vi "Main.vi"(11 "Module Admin":refnum<class "Delacor_lib_QMH_Module Admin.lvclass">) -> ()   [LabVIEW 2020, in "Configuration.lvlib"]
doc: "This template is based off of the Queued Message Handler design pattern and the Queued Message Handler project template that ships with LabVIEW.\n\nThe main difference is that the queue is private to this module and communication between modules is performed via Broadcast and Request events.\n\nRequest events are wrapped in public API methods and are handled in the Event Handling Loop (EHL) of this VI. Any module can register for Broadcast events sent by this module. The EHL generates messages based on user interface actions.\n\nThe Message Handling Loop (MHL) processes messages generated by the EHL, or by other messages. The messages are string values, so new messages can be added easily to the Message Cases case structure in the MHL. Each message cluster can also provide an optional value for Message Data, which is a variant that can be converted to whatever message-specific data is required.\n_____\nBased on Delacor QMH Project Template 5.0.0.82."
uses:
  Configuration.lvlib
  <vilib>/Delacor/Delacor QMH/Libraries/Module Admin_class/Delacor_lib_QMH_Module Admin.lvclass
  Module Data--cluster.ctl
  Stop Argument--cluster.ctl
  <vilib>/Delacor/Delacor QMH/Libraries/Message Queue_class/Delacor_lib_QMH_Message Queue.lvclass/Delacor_lib_QMH_Message Queue.ctl
  SQLITE Inventory/Invetory Data Type.ctl
  <vilib>/Utility/miscctls.llb/LVPointTypeDef.ctl
  <vilib>/Delacor/Delacor QMH/Libraries/Module Admin_class/Delacor_lib_QMH_Module Admin.lvclass/Delacor_lib_QMH_Module Admin.ctl
  TypeDefinitions/CurrencyEnum.ctl
  <vilib>/Delacor/Delacor QMH/Libraries/Message Queue_class/Delacor_lib_QMH_Enqueue Message (Single).vi
  <vilib>/Delacor/Delacor QMH/Libraries/Module Admin_class/Delacor_lib_QMH_Get External Launch.vi
  <vilib>/Utility/error.llb/Error Cluster From Error Code.vi
  <vilib>/ErrorRing/Error Ring.xnode
  <vilib>/Delacor/Delacor QMH/Libraries/Message Queue_class/Delacor_lib_QMH_Message Queue.lvclass
  SQLITE Inventory/SQLITE Inventory.lvlib
  Product Selecting Pane/Product Selecting Pane.lvlib
  Money Control Pane/Money Control Pane.lvlib
  Config Files Management/Config File Management.lvlib
panel:
  in  "Change Currency":bool
  in  "Coin Management":T1
  in  "Inventory Management":T2(tab)
  in  "Add Product":bool
  in  "Quantity":dbl
  in  "Price":dbl
  in  "Product Name":string
  in  "Change Stock":bool
  in  "Add to stock":bool
  in  "Stock":u32
  in  "Product UI":u16(ring) items=["Cheetos", "Cheetos Puff", "Doritos 3D", "Doritos Incognita", "Doritos Nacho", "Gomilokas", "Takis Verde"]
  in  "Update all price":bool
  in  "Convertion Ratio":dbl
  in  "Update single price":bool
  in  "New Price":dbl
  in  "Product UP":u16(ring) items=["Cheetos", "Cheetos Puff", "Doritos 3D", "Doritos Incognita", "Doritos Nacho", "Gomilokas", "Takis Verde"]
  in  "Product D":u16(ring) items=["Cheetos", "Cheetos Puff", "Doritos 3D", "Doritos Incognita", "Doritos Nacho", "Gomilokas", "Takis Verde"]
  in  "Delete":bool
  out "error out":errorcluster
  # "General Settings"
  # "1 of old currency is equal to"
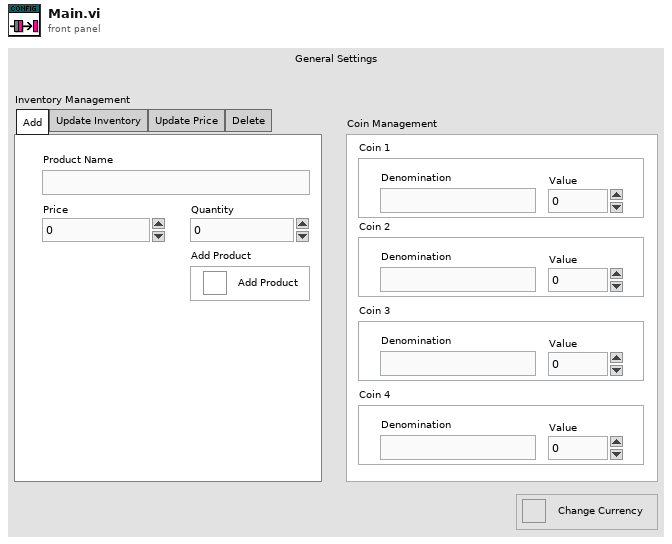
[diagram p1: front panel]
types:
  T1 = cluster{"Coin 1":cluster{"Denomination":string, "Value":dbl}, "Coin 2":cluster{"Denomination":string, "Value":dbl}, "Coin 3":cluster{"Denomination":string, "Value":dbl}, "Coin 4":cluster{"Denomination":string, "Value":dbl}}
  T2 = enum32{"Add", "Update Inventory", "Update Price", "Delete"}
  T3 = typedef "Configuration.lvlib/Request Events--cluster.ctl" = cluster{"Stop Module":refnum<user-event>, "Show Panel":refnum<user-event>, "Hide Panel":refnum<user-event>, "Get Module Execution Status":refnum<user-event>, "Show Diagram":refnum<user-event>}
  T4 = typedef "Configuration.lvlib/Module Data--cluster.ctl" = cluster{"Status":string, "Products":string[], "Ref Array":refnum<vi>[], "Product UI":string, "Product UP":string, "Product D":string, "Stock":u32}
  T5 = enum32{"invalid lock state", "Not Locked", "Locked (No Password)", "Password-protected"}
  T6 = typedef "Configuration.lvlib/Stop Argument--cluster.ctl" = cluster{"Origin":string, "Exit via Stop Module Req?":bool, "Wait for Module to stop?":bool}
  T7 = typedef "Invetory Data Type.ctl" = cluster{"Name":string, "Price":dbl, "Stock":dbl}
  T8 = typedef "LVPointTypeDef.ctl" = cluster{"Horizontal":i16, "Vertical":i16}
  T9 = enum32{"Invalid", "Standard", "Closed", "Hidden", "Minimized", "Maximized"}
  T10 = typedef "CurrencyEnum.ctl" = enum16{"USD", "MXN", "EUR", "GBP"}
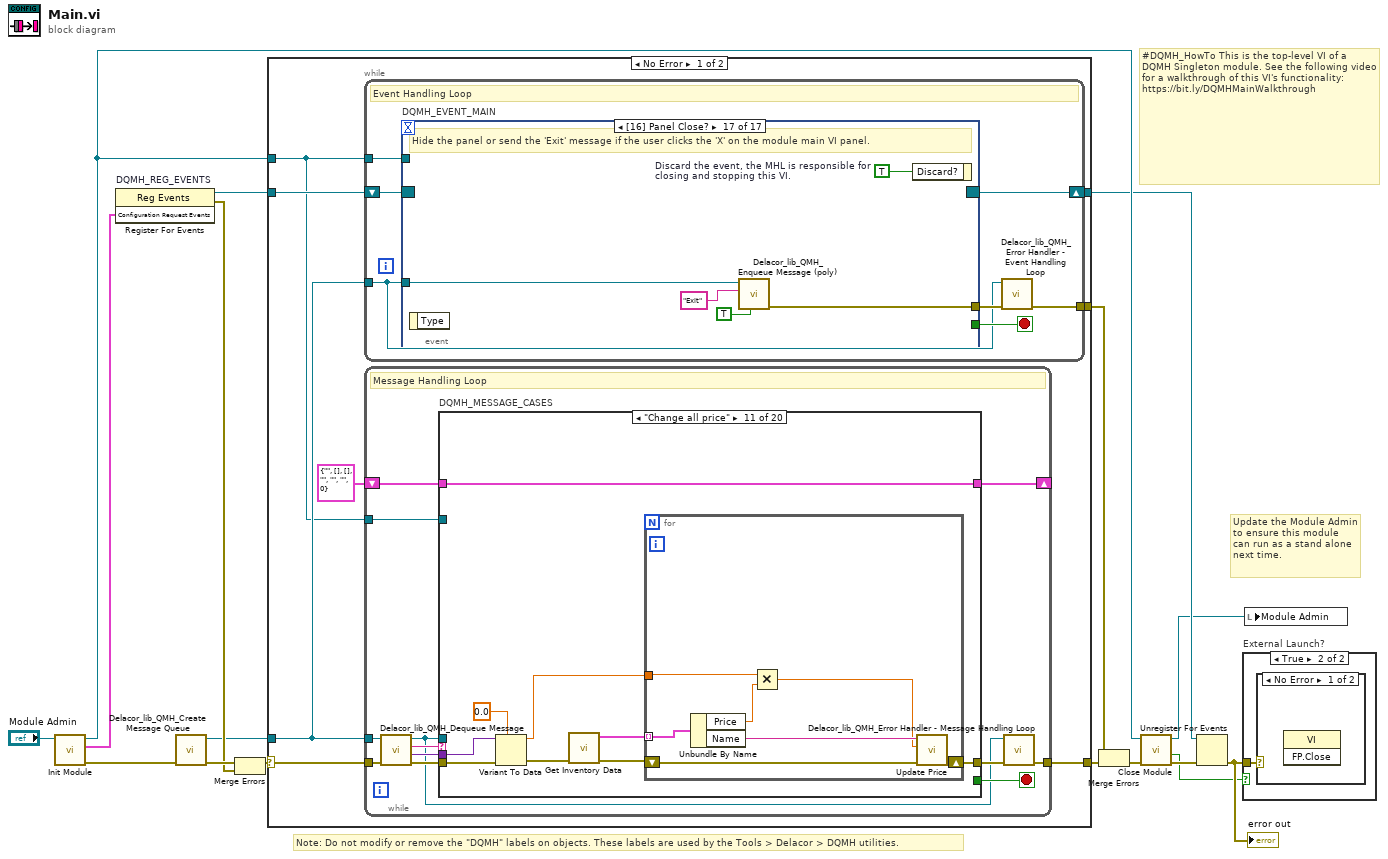
[diagram p0: block diagram]
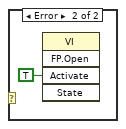
[diagram p3: hidden frame]
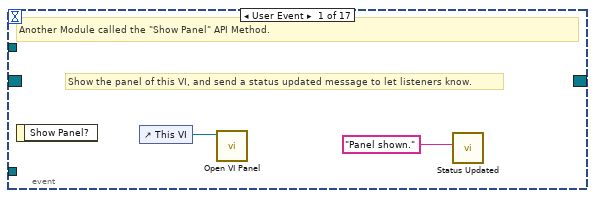
[diagram p4: hidden frame]
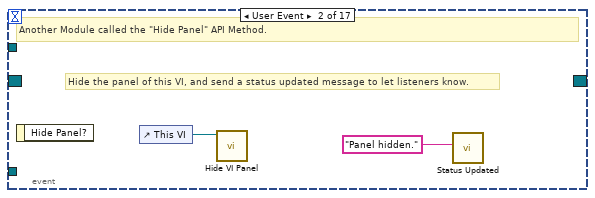
[diagram p5: hidden frame]
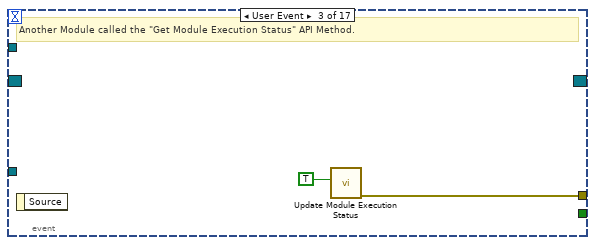
[diagram p6: hidden frame]
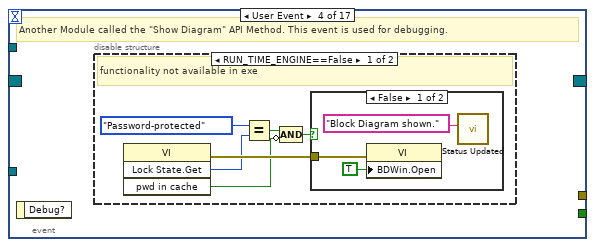
[diagram p7: hidden frame]
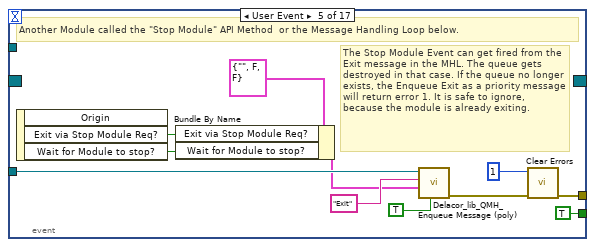
[diagram p10: hidden frame]
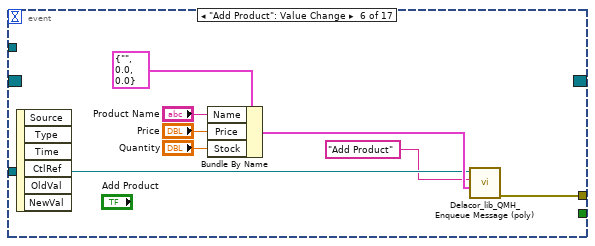
[diagram p11: hidden frame]
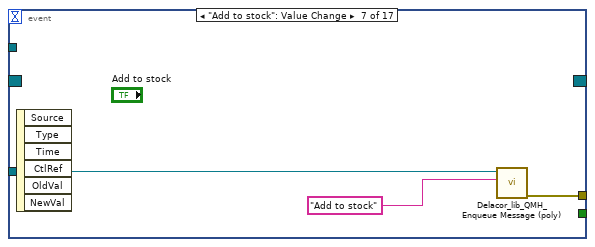
[diagram p12: hidden frame]
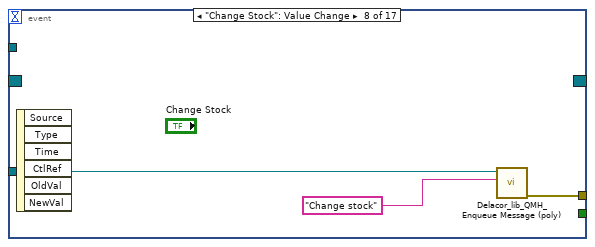
[diagram p13: hidden frame]
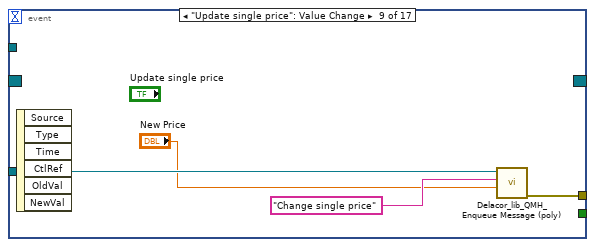
[diagram p14: hidden frame]
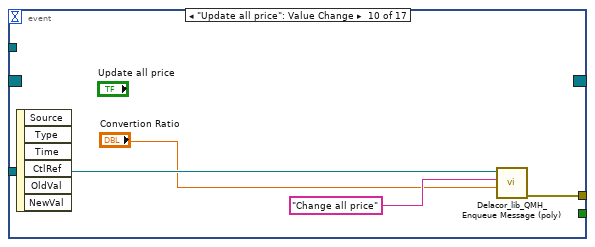
[diagram p15: hidden frame]
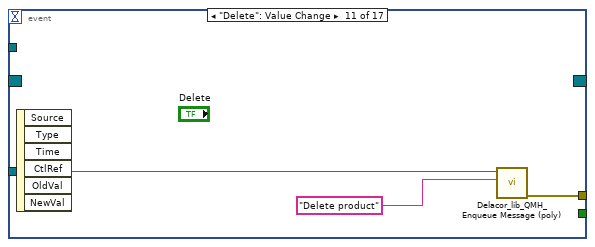
[diagram p16: hidden frame]
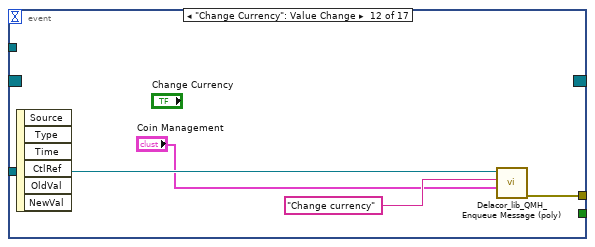
[diagram p17: hidden frame]
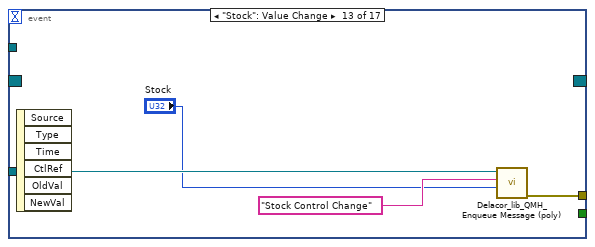
[diagram p18: hidden frame]
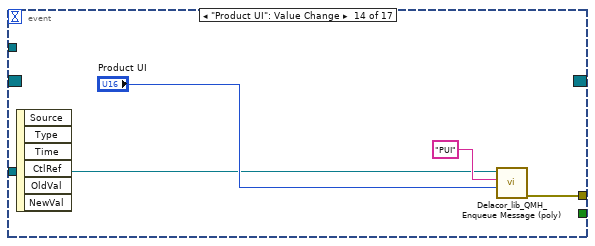
[diagram p19: hidden frame]
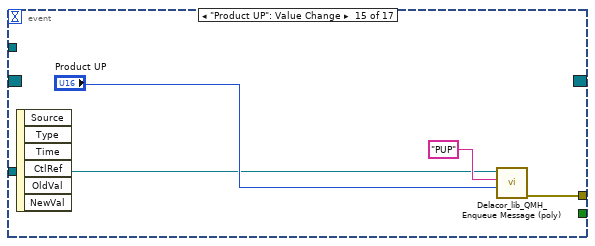
[diagram p20: hidden frame]
diagram:
  # "#DQMH_HowTo This is the top-level VI of a DQMH Singleton module. See the following video for a walkthrough of this VI's functionality: https://bit.ly/DQMHMainWalkthrough"
  # "Note: Do not modify or remove the \"DQMH\" labels on objects. These labels are used by the Tools > Delacor > DQMH utilities."
  # "Update the Module Admin to ensure this module can run as a stand alone next time."
  n1 = call "Init Module.vi"("Singleton Module Admin in"="Module Admin") -> ("error out"=w16:errorcluster, "Configuration Request Events"=w5:T3, "Singleton Module Admin out"=w8:refnum<class "Delacor_lib_QMH_Module Admin.lvclass">)  [unwired: 8 in]
  n2 = register-events "DQMH_REG_EVENTS"(w5) -> (reference out=w6:refnum<event-registration>, error out=w9:errorcluster)  [unwired: 2 in]
  n3 = call <vilib>:"Delacor_lib_QMH_Create Message Queue.vi"("error in (no error)"=w16) -> ("error out"=w11:errorcluster, "Message Queue"=w4:refnum<class "Delacor_lib_QMH_Message Queue.lvclass">)  [unwired: 9 in]
  n4 = Merge Errors(w11, w9) -> (w10:errorcluster)
  n5 = case shown="No Error" w10 {
    selector: w10 -> [w23 w329]
    tunnel: [w25 w328] -> w17
    tunnel: [w22 w334] -> w7
    tunnel: w6 -> [w20 w334]
    tunnel: w4 -> [w19 w327]
    tunnel: [w24 _] -> w14
    tunnel: w8 -> [w18 w330]
    frame No Error {
      n6 = while {
        tunnel: w19 -> [w26]
        shift-right: [w29] -> w22
        shift-left: w20 -> [w30]
        tunnel: [w31] -> w24
        tunnel: w18 -> [w27]
        stop <- w28 stop-if-true
        # "Event Handling Loop"
        n7 = event "DQMH_EVENT_MAIN" shown="[16] Panel Close?" {
          selector: w30 -> [_ _ _ _ _ _ _ _ _ _ _ _ _ _ _ _ _]
          dyn-events: [_ _ _ _ _ _ _ _ _ _ _ _ _ _ _ _ _] -> w29
          timeout: _ -> [_ _ _ _ _ _ _ _ _ _ _ _ _ _ _ _ _]
          tunnel: [_ _ _ _ TRUE ("Discard?") _ _ _ _ _ _ _ _ _ _ _ _] -> w28
          tunnel: w26 -> [_ _ _ _ w54 w60 w67 w70 w74 w78 w81 w85 w89 w92 w96 w100 w106]
          tunnel: [_ _ w38 _ w57 w66 w69 w72 w76 w80 w83 w87 w91 w95 w99 w103 w108] -> w32
          tunnel: w27 -> [_ _ _ _ _ _ _ _ _ _ _ _ _ _ _ _ _]
          event User Event {
            # "Show the panel of this VI, and send a status updated message to let listeners know."
            # "Another Module called the \"Show Panel\" API Method."
            n8 = event-data() -> ()  [unwired: 1 in, 1 out]
            n9 = control-ref of="This VI"() -> (w34:refnum<vi>)
            n10 = call "Open VI Panel.vi"("VI"=w34) -> ()  [unwired: 10 in, 1 out]
            n11 = call "Status Updated.vi"("Status"="Panel shown." ("format string")) -> ()  [unwired: 10 in, 1 out]
          }
          event User Event {
            # "Hide the panel of this VI, and send a status updated message to let listeners know."
            # "Another Module called the \"Hide Panel\" API Method."
            n12 = event-data() -> ()  [unwired: 1 in, 1 out]
            n13 = control-ref of="This VI"() -> (w36:refnum<vi>)
            n14 = call "Hide VI Panel.vi"("VI"=w36) -> ()  [unwired: 10 in, 1 out]
            n15 = call "Status Updated.vi"("Status"="Panel hidden." ("format string")) -> ()  [unwired: 10 in, 1 out]
          }
          event User Event {
            # "Another Module called the \"Get Module Execution Status\" API Method."
            n16 = event-data() -> ()  [unwired: 1 in, 1 out]
            n17 = call "Update Module Execution Status.vi"("Running?"=TRUE) -> ("error out"=w38:errorcluster)  [unwired: 10 in]
          }
          event User Event {
            # "Another Module called the \"Show Diagram\" API Method. This event is used for debugging."
            n18 = event-data() -> ()  [unwired: 1 in, 1 out]
            n19 = disable-structure shown="RUN_TIME_ENGINE==False" {
              frame condition #0 (active) {
                # "functionality not available in exe"
                n20 = invoke class="VI" method="Lock State.Get"() -> (error out=w44:errorcluster, "Get Lock State"=w43:T5, "pwd in cache"=w40:bool)  [unwired: 4 in, 1 out]
                n21 = Equal?(x=T5."Password-protected", y=w43) -> (x = y?=w41:bool)
                n22 = Compound Arithmetic op=AND(w41, invert w40) -> (w39:bool)
                n23 = case shown="False" w39 {
                  tunnel: w44 -> [w47 _]
                  frame False {
                    n24 = property class="VI"(error in=w47, "BDWin.Open"=TRUE ("Block Diagram Window:Open")) -> ()  [unwired: 1 in, 2 out]
                    n25 = call "Status Updated.vi"("Status"="Block Diagram shown." ("format string")) -> ()  [unwired: 10 in, 1 out]
                  }
                  frame True {
                    # "Password-protected VI, and the password is not in the cache. Do not show the diagram."
                  }
                }
              }
              frame condition #1 {
              }
            }
          }
          event User Event {
            # "The Stop Module Event can get fired from the Exit message in the MHL. The queue gets destroyed in that case. If the queue no longer exists, the Enqueue Exit as a priority message will return error 1. It is safe to ignore, because the module is already exiting."
            # "Another Module called the \"Stop Module\" API Method  or the Message Handling Loop below."
            n26 = event-data() -> ("Exit via Stop Module Req?"=w50:bool, "Wait for Module to stop?"=w49:bool)  [unwired: 1 in, 1 out]
            n27 = Bundle By Name(cluster=T6 {"Origin"="", "Exit via Stop Module Req?"=FALSE, "Wait for Module to stop?"=FALSE} ("Stop Argument"), "Exit via Stop Module Req?"=w50, "Wait for Module to stop?"=w49) -> (w48:T6)
            n28 = call-poly <vilib>:"Delacor_lib_QMH_Enqueue Message (poly).vi"("Priority Message? (F)"=TRUE, "Message Data"=w48, "Message"="Exit", "Message Queue in"=w54) -> ("error out"=w58:errorcluster)  [unwired: 6 in, 1 out]
            n29 = call <vilib>:"Clear Errors.vi"("error in (no error)"=w58, "specific error code to clear (0: all)"=1) -> ("error out"=w57:errorcluster)  [unwired: 4 in, 1 out]
          }
          event "Add Product": Value Change {
            n30 = event-data() -> ()  [unwired: 1 in, 6 out]
            n31 = Bundle By Name(cluster=T7 {"Name"="", "Price"=0.0, "Stock"=0.0} ("Cluster"), "Name"="Product Name", "Price"="Price", "Stock"="Quantity") -> (w61:T7)
            n32 = call-poly <vilib>:"Delacor_lib_QMH_Enqueue Message (poly).vi"("Message Data"=w61, "Message"="Add Product", "Message Queue in"=w60) -> ("error out"=w66:errorcluster)  [unwired: 7 in, 1 out]
          }
          event "Add to stock": Value Change {
            n33 = event-data() -> ()  [unwired: 1 in, 6 out]
            n34 = call-poly <vilib>:"Delacor_lib_QMH_Enqueue Message (poly).vi"("Message"="Add to stock", "Message Queue in"=w67) -> ("error out"=w69:errorcluster)  [unwired: 8 in, 1 out]
          }
          event "Change Stock": Value Change {
            n35 = event-data() -> ()  [unwired: 1 in, 6 out]
            n36 = call-poly <vilib>:"Delacor_lib_QMH_Enqueue Message (poly).vi"("Message"="Change stock", "Message Queue in"=w70) -> ("error out"=w72:errorcluster)  [unwired: 8 in, 1 out]
          }
          event "Update single price": Value Change {
            n37 = event-data() -> ()  [unwired: 1 in, 6 out]
            n38 = call-poly <vilib>:"Delacor_lib_QMH_Enqueue Message (poly).vi"("Message Data"="New Price", "Message"="Change single price", "Message Queue in"=w74) -> ("error out"=w76:errorcluster)  [unwired: 7 in, 1 out]
          }
          event "Update all price": Value Change {
            n39 = event-data() -> ()  [unwired: 1 in, 6 out]
            n40 = call-poly <vilib>:"Delacor_lib_QMH_Enqueue Message (poly).vi"("Message Data"="Convertion Ratio", "Message"="Change all price", "Message Queue in"=w78) -> ("error out"=w80:errorcluster)  [unwired: 7 in, 1 out]
          }
          event "Delete": Value Change {
            n41 = event-data() -> ()  [unwired: 1 in, 6 out]
            n42 = call-poly <vilib>:"Delacor_lib_QMH_Enqueue Message (poly).vi"("Message"="Delete product", "Message Queue in"=w81) -> ("error out"=w83:errorcluster)  [unwired: 8 in, 1 out]
          }
          event "Change Currency": Value Change {
            n43 = event-data() -> ()  [unwired: 1 in, 6 out]
            n44 = call-poly <vilib>:"Delacor_lib_QMH_Enqueue Message (poly).vi"("Message Data"="Coin Management", "Message"="Change currency", "Message Queue in"=w85) -> ("error out"=w87:errorcluster)  [unwired: 7 in, 1 out]
          }
          event "Stock": Value Change {
            n45 = event-data() -> ()  [unwired: 1 in, 6 out]
            n46 = call-poly <vilib>:"Delacor_lib_QMH_Enqueue Message (poly).vi"("Message Data"="Stock", "Message"="Stock Control Change", "Message Queue in"=w89) -> ("error out"=w91:errorcluster)  [unwired: 7 in, 1 out]
          }
          event "Product UI": Value Change {
            n47 = event-data() -> ()  [unwired: 1 in, 6 out]
            n48 = call-poly <vilib>:"Delacor_lib_QMH_Enqueue Message (poly).vi"("Message Data"="Product UI", "Message"="PUI", "Message Queue in"=w92) -> ("error out"=w95:errorcluster)  [unwired: 7 in, 1 out]
          }
          event "Product UP": Value Change {
            n49 = event-data() -> ()  [unwired: 1 in, 6 out]
            n50 = call-poly <vilib>:"Delacor_lib_QMH_Enqueue Message (poly).vi"("Message Data"="Product UP", "Message"="PUP", "Message Queue in"=w96) -> ("error out"=w99:errorcluster)  [unwired: 7 in, 1 out]
          }
          event "Product D": Value Change {
            n51 = event-data() -> ()  [unwired: 1 in, 6 out]
            n52 = call-poly <vilib>:"Delacor_lib_QMH_Enqueue Message (poly).vi"("Message Data"="Product D", "Message"="PD", "Message Queue in"=w100) -> ("error out"=w103:errorcluster)  [unwired: 7 in, 1 out]
          }
          event Panel Close? {
            w107 = TRUE  # Discard the event, the MHL is responsible for closing and stopping this VI.
            # "Hide the panel or send the 'Exit' message if the user clicks the 'X' on the module main VI panel."
            n53 = event-data() -> ()  [unwired: 1 in, 1 out]
            n54 = call-poly <vilib>:"Delacor_lib_QMH_Enqueue Message (poly).vi"("Priority Message? (F)"=TRUE, "Message"="Exit", "Message Queue in"=w106) -> ("error out"=w108:errorcluster)  [unwired: 7 in, 1 out]
            n55 = event-data("Discard?"=w107) -> ()  [unwired: 1 in, 1 out]
          }
        }
        n56 = call-dynamic "Delacor_lib_QMH_Error Handler - Event Handling Loop.vi"("error in (no error)"=w32, "Message Queue in"=w26) -> ("dup error in"=w31:errorcluster)  [unwired: 8 in, 1 out]
      }
      n57 = while {
        tunnel: w19 -> [w111]
        shift-right: [w115] -> _
        shift-left: T4 {"Status"="", "Products"=[], "Ref Array"=[], "Product UI"="", "Product UP"="", "Product D"="", "Stock"=0} ("Data Cluster") -> [w116]
        tunnel: w23 -> [w119]
        tunnel: [w117] -> w25
        tunnel: w18 -> [w109]
        stop <- w114 stop-if-true
        # "Message Handling Loop"
        n58 = call-dynamic "Delacor_lib_QMH_Dequeue Message.vi"("error in (no error)"=w119, "Message Queue in"=w111) -> ("error out"=w118:errorcluster, "Message Data"=w112:variant, "Message"=w113:string, "Message Queue out"=w110:refnum<class "Delacor_lib_QMH_Message Queue.lvclass">)  [unwired: 6 in]
        n59 = case "DQMH_MESSAGE_CASES" shown="\"Change all price\"" w113 {
          selector: w113 -> [_ _ _ _ _ _ _ _ _ _ _ _ _ _ _ _ _ _ _ w314]
          tunnel: w110 -> [w125 _ _ _ _ _ _ _ _ _ _ _ w245 _ _ _ _ w283 w306 _]
          tunnel: w118 -> [w145 w153 w167 w176 w185 w187 w199 w207 w210 w221 w229 w244 w254 w262 w265 w267 w272 w290 w312 w316]
          tunnel: [w127 w152 w166 w175 w184 w186 w198 w206 w211 w214 w223 w242 w247 w262 w264 w267 w271 w286 w309 w317] -> w120
          tunnel: w116 -> [w135 w151 w161 w170 w179 w195 w200 w208 w212 w220 w230 w243 w253 w261 w263 w266 w269 w285 w305 w315]
          tunnel: [w134 w149 w164 w173 w182 w195 w200 w208 w212 w220 w230 w239 w253 w261 w263 w266 w269 w285 w305 w315] -> w115
          tunnel: [_ _ _ _ _ _ _ _ _ _ _ _ _ _ _ _ _ _ w304 _] -> w114
          tunnel: w112 -> [_ _ w165 w174 w183 _ _ w203 _ w218 w228 w241 w252 _ _ _ _ w284 w303 _]
          tunnel: w109 -> [w136 _ _ _ _ _ _ _ _ _ _ _ _ _ _ _ _ w282 w298 _]
          frame "Initialize" {
            # "Initialize - Any operation that needs to be done before the module can receive messages. Synchronize Caller Events.vi will inform Start Module.vi that the module has launched and is ready to receive messages. Module Did Init.vi will broadcast that the module initialized."
            n60 = call "Synchronize Caller Events.vi"("error in (no error)"=w145, "Singleton Module Admin in"=w136) -> ("error out"=w144:errorcluster, "Singleton Module Admin out"=w131:refnum<class "Delacor_lib_QMH_Module Admin.lvclass">)  [unwired: 8 in]
            n61 = property class="Module Admin"(reference=w131) -> ("Accessors:External Launch"=w140:bool)  [unwired: 1 in, 2 out]
            n62 = control-ref of="Product D"() -> (w124:refnum<vi>)
            n63 = control-ref of="Product UP"() -> (w123:refnum<vi>)
            n64 = control-ref of="Product UI"() -> (w122:refnum<vi>)
            n65 = Build Array(w124, w123, w122) -> (w121:refnum<vi>[])
            n66 = Select(t=T9."Hidden" ("State"), s=w140, f=T9."Standard" ("State")) -> (s? t:f=w137:T9)
            n67 = call "Module Name--constant.vi"() -> ("Module Name"=w132:string)  [unwired: 11 in]
            n68 = call "Module Name--constant.vi"() -> ("Module Name"=w143:string)  [unwired: 11 in]
            n69 = call "Module Did Init.vi"("error in (no error)"=w144, "Initialized?"=TRUE, "Origin"=w132) -> ("error out"=w128:errorcluster)  [unwired: 8 in]
            n70 = property class="VI"("Front Panel.Title"=w143) -> (reference out=w142:refnum<vi>, error out=w147:errorcluster)  [unwired: 2 in]
            n71 = invoke class="VI" method="FP.Open"(reference=w142, error in=w147, "State"=w137) -> (reference out=w141:refnum<vi>, error out=w146:errorcluster)  [unwired: 2 in, 3 out]
            n72 = Bundle By Name(cluster=w135, "Status"="Initial Message" ("Initial Message"), "Ref Array"=w121) -> (w134:T4)
            n73 = call-poly <vilib>:"Delacor_lib_QMH_Enqueue Message (poly).vi"("error in (no error)"=w128, "Message"="Update DB", "Message Queue in"=w125) -> ("error out"=w127:errorcluster)  [unwired: 7 in, 1 out]
            n74 = invoke class="VI" method="FP.Center"(reference=w141, error in=w146) -> ()  [unwired: 1 in, 3 out]
            n75 = property on="Pane" class="Pane"("Origin"=T8 {"Horizontal"=0, "Vertical"=0}) -> ()  [unwired: 2 in, 2 out]
          }
          frame "Update DB" {
            # "Update product Controls when DB products has been modified"
            n76 = call "Get Inventory Data.vi"("error in (no error)"=w153) -> ("error out"=w152:errorcluster, "Array"=w154:T7[])  [unwired: 9 in]
            n77 = Unbundle By Name(w151) -> ("Ref Array"=w150:refnum<vi>[])
            n78 = for {
              tunnel: w154 -> [w158] mode=indexing
              tunnel: [w157] -> w148 mode=indexing
              n79 = Unbundle By Name(w158) -> ("Name"=w157:string)
            }
            n80 = for {
              tunnel: w148 -> [w156]
              tunnel: w150 -> [w155] mode=indexing
              n81 = property class="Ring (strict)"(reference=w155, "Strings []"=w156) -> ()  [unwired: 1 in, 2 out]
            }
            n82 = Bundle By Name(cluster=w151, "Products"=w148) -> (w149:T4)
          }
          frame "PUI" {
            n83 = Variant To Data(error in=w167, type=u16 0, Variant=w165) -> (data=w162:u16, error out=w166:errorcluster)
            n84 = Unbundle By Name(w161) -> ("Products"=w160:string[])
            n85 = Index Array(array=w160, index=w162) -> (element=w159:string)
            n86 = Bundle By Name(cluster=w161, "Product UI"=w159) -> (w164:T4)
          }
          frame "PUP" {
            n87 = Variant To Data(error in=w176, type=u16 0, Variant=w174) -> (data=w171:u16, error out=w175:errorcluster)
            n88 = Unbundle By Name(w170) -> ("Products"=w169:string[])
            n89 = Index Array(array=w169, index=w171) -> (element=w168:string)
            n90 = Bundle By Name(cluster=w170, "Product UP"=w168) -> (w173:T4)
          }
          frame "PD" {
            n91 = Variant To Data(error in=w185, type=u16 0, Variant=w183) -> (data=w180:u16, error out=w184:errorcluster)
            n92 = Unbundle By Name(w179) -> ("Products"=w178:string[])
            n93 = Index Array(array=w178, index=w180) -> (element=w177:string)
            n94 = Bundle By Name(cluster=w179, "Product D"=w177) -> (w182:T4)
          }
          frame "Add to stock" {
            n95 = Unbundle By Name(w195) -> ("Product UI"=w194:string, "Stock"=w190:u32)
            n96 = call "Get Product Info.vi"("error in (no error)"=w187, "Name"=w194) -> ("error out"=w188:errorcluster, "Product Info"=w193:T7)  [unwired: 7 in, 1 out]
            n97 = Unbundle By Name(w193) -> ("Name"=w192:string, "Stock"=w191:dbl)
            n98 = Add(x=w191, y=w190) -> (x+y=w189:dbl)
            n99 = call "Update Stock.vi"("error in (no error)"=w188, "Stock"=w189, "Name"=w192) -> ("error out"=w186:errorcluster)  [unwired: 8 in]
          }
          frame "Change stock" {
            n100 = Unbundle By Name(w200) -> ("Product UI"=w196:string, "Stock"=w197:u32)
            n101 = call "Update Stock.vi"("error in (no error)"=w199, "Stock"=w197, "Name"=w196) -> ("error out"=w198:errorcluster)  [unwired: 8 in]
          }
          frame "Change single price" {
            n102 = Unbundle By Name(w208) -> ("Product UP"=w205:string)
            n103 = Variant To Data(error in=w207, type=0.0 ("New Price"), Variant=w203) -> (data=w201:dbl, error out=w204:errorcluster)
            n104 = call "Update Price.vi"("error in (no error)"=w204, "Price"=w201, "Name"=w205) -> ("error out"=w206:errorcluster)  [unwired: 8 in]
          }
          frame "Delete product" {
            n105 = Unbundle By Name(w212) -> ("Product D"=w209:string)
            n106 = call "Delete Product.vi"("error in (no error)"=w210, "Name"=w209) -> ("error out"=w211:errorcluster)  [unwired: 9 in]
          }
          frame "Change currency" {
            n107 = Variant To Data(error in=w221, type=T1 {"Coin 1"={"Denomination"="", "Value"=0.0}, "Coin 2"={"Denomination"="", "Value"=0.0}, "Coin 3"={"Denomination"="", "Value"=0.0}, "Coin 4"={"Denomination"="", "Value"=0.0}} ("Coin Management"), Variant=w218) -> (data=w216:T1, error out=w219:errorcluster)
            n108 = Cluster To Array(cluster=w216) -> (array=w215:cluster{"Denomination":string, "Value":dbl}[])
            n109 = call "Change Currency.vi"("Coin"=w215) -> ("error out"=w213:errorcluster)  [unwired: 10 in]
            n110 = Merge Errors(w213, w219) -> (w214:errorcluster)
          }
          frame "Change all price" {
            n111 = Variant To Data(error in=w229, type=0.0 ("New Price"), Variant=w228) -> (data=w222:dbl, error out=w225:errorcluster)
            n112 = call "Get Inventory Data.vi"("error in (no error)"=w225) -> ("error out"=w224:errorcluster, "Array"=w226:T7[])  [unwired: 9 in]
            n113 = for {
              tunnel: w226 -> [w235] mode=indexing
              shift-right: [w236] -> w223
              shift-left: w224 -> [w237]
              tunnel: w222 -> [w232]
              n114 = Unbundle By Name(w235) -> ("Price"=w233:dbl, "Name"=w234:string)
              n115 = Multiply(x=w232, y=w233) -> (x*y=w231:dbl)
              n116 = call "Update Price.vi"("error in (no error)"=w237, "Price"=w231, "Name"=w234) -> ("error out"=w236:errorcluster)  [unwired: 8 in]
            }
          }
          frame "Stock Control Change" {
            n117 = Variant To Data(error in=w244, type=u32 0 ("Stock"), Variant=w241) -> (data=w238:u32, error out=w242:errorcluster)
            n118 = Bundle By Name(cluster=w243, "Stock"=w238) -> (w239:T4)
          }
          frame "Add Product" {
            # "Add Product Button has been pushed, product is added to Data Base. If the products exists, a dialog will be shown warning the user."
            n119 = Variant To Data(error in=w254, type=T7 {"Name"="", "Price"=0.0, "Stock"=0.0} ("Cluster"), Variant=w252) -> (data=w249:T7, error out=w250:errorcluster)
            n120 = call "Set New Product.vi"("error in (no error)"=w250, "Cluster"=w249) -> ("error out"=w246:errorcluster, "success?"=w248:bool)  [unwired: 6 in]
            n121 = case shown="False" w248 {
              tunnel: [w255 w260] -> w247
              tunnel: w246 -> [w255 w259]
              tunnel: w245 -> [_ w257]
              frame False {
                n122 = One Button Dialog(message="The product you tried to add already exists.") -> ()  [unwired: 1 in, 1 out]
              }
              frame True {
                n123 = call-poly <vilib>:"Delacor_lib_QMH_Enqueue Message (poly).vi"("error in (no error)"=w259, "Message"="Update DB", "Message Queue in"=w257) -> ("error out"=w260:errorcluster)  [unwired: 7 in, 1 out]
              }
            }
          }
          frame "--- Module Specific ---" {
            # "Separator -- The following cases handle messages specific to this Module."
          }
          frame "---Copy This Frame---" {
            # "Duplicate this frame when creating new messages.  Change this comment in the duplicated frame to describe this message."
            n124 = Merge Errors(w265) -> (w264:errorcluster)
          }
          frame "--- Exit and Error Handling---" {
            # "Separator - The following cases handle errors and exit messages."
          }
          frame "Simulate MHL Error" {
            # "#DQMH_HowTo The 'Simulate MHL Error' button  illustrates how the MHL handles errors. This event is instructional in nature and can be removed."
            # "Simulate an error occurring at the MHL"
            n125 = call "Module Name--constant.vi"() -> ("Module Name"=w268:string)  [unwired: 11 in]
            n126 = xnode "Error Ring"("parameter 0"=w268) -> ("error out"=w270:errorcluster)
            n127 = Merge Errors(w272, w270) -> (w271:errorcluster)
          }
          frame "Error" {
            # "#CodeRecommended - If you ever change the name of this \"Error\" message, you'll need to update the name in the Check Loop Error.vi as well."
            # "#CodeRecommended - If the module is running in standalone mode (External Launch = FALSE), this code will pop up an error dialog and call the 'Exit' message if an error occurs. Add more fine-grained error handling here."
            # "Error - Check the error message data and respond accordingly. This message is sent by the \"Error Handler\" VIs at the end of each loop in this application."
            n128 = property class="Module Admin"(reference=w282) -> ("Accessors:External Launch"=w281:bool)  [unwired: 1 in, 2 out]
            n129 = Variant To Data(error in=w290, type=errorcluster {"status"=FALSE, "code"=0, "source"=""} ("error constant"), Variant=w284) -> (data=w291:errorcluster, error out=w288:errorcluster)
            n130 = call "Module Name--constant.vi"() -> ("Module Name"=w280:string)  [unwired: 11 in]
            n131 = call "Error Reported.vi"("Additional Information"=w280, "Error"=w291) -> ()  [unwired: 9 in, 1 out]
            n132 = case shown="False" w281 {
              tunnel: [w296 _] -> w287
              tunnel: w283 -> [w294 _]
              tunnel: w291 -> [w295 _]
              frame False {
                # "If the module is running standalone, then pop up an error dialog and call the \"Exit\" message."
                n133 = call <vilib>:"Simple Error Handler.vi"("error in (no error)"=w295) -> ()  [unwired: 4 in, 5 out]
                n134 = call-poly <vilib>:"Delacor_lib_QMH_Enqueue Message (poly).vi"("Priority Message? (F)"=TRUE, "Message"="Exit", "Message Queue in"=w294) -> ("error out"=w296:errorcluster)  [unwired: 7 in, 1 out]
              }
              frame True {
                # "If the module was launched externally, calling the Error Reported broadcast VI is the only action performed by the \"Error\" message. The module's caller can then process the error appropriately."
              }
            }
            n135 = Merge Errors(w288, w287) -> (w286:errorcluster)
            n136 = local write "error out"(w286) -> ()
          }
          frame "Exit" {
            w302 = 91  # 91: not all Exit messages will have an argument
            w304 = TRUE  # Stop the VI
            # "Release the message queue reference"
            # "#CodeNeeded - Add any required cleanup code here"
            # "Exit - Exit the application."
            n137 = Variant To Data(error in=w312, type=T6 {"Origin"="", "Exit via Stop Module Req?"=FALSE, "Wait for Module to stop?"=FALSE} ("Stop Argument"), Variant=w303) -> (data=w300:T6, error out=w308:errorcluster)
            n138 = call <vilib>:"Clear Errors.vi"("error in (no error)"=w308, "specific error code to clear (0: all)"=w302) -> ("error out"=w311:errorcluster)  [unwired: 4 in, 1 out]
            n139 = control-ref of="This VI"() -> (w299:refnum<vi>)
            n140 = call-dynamic "Delacor_lib_QMH_Release Message Queue.vi"("error in (no error)"=w311, "Message Queue"=w306) -> ("error out"=w310:errorcluster)  [unwired: 9 in]
            n141 = call "Handle Exit.vi"("Stop Argument"=w300, "Admin in"=w298, "VI reference"=w299) -> ("error out"=w307:errorcluster)  [unwired: 7 in, 1 out]
            n142 = Merge Errors(w310, w307) -> (w309:errorcluster)
            n143 = call "Configuration Change.vi"("Enum"=CurrencyEnum."USD") -> ()  [unwired: 10 in, 1 out]
            n144 = call "Update Products.vi"() -> ()  [unwired: 11 in, 1 out]
          }
          frame Default {
            # "'Default' case only runs if there is a message that isn't defined in any of the other cases.  Output a programming error."
            n145 = call "Module Name--constant.vi"() -> ("Module Name"=w313:string)  [unwired: 11 in]
            n146 = xnode "Error Ring"("parameter 0"=w314, "parameter 1"=w313) -> ("error out"=w318:errorcluster)
            n147 = Merge Errors(w316, w318) -> (w317:errorcluster)
          }
        }
        n148 = call-dynamic "Delacor_lib_QMH_Error Handler - Message Handling Loop.vi"("error in (no error)"=w120, "Message Queue in"=w110) -> ("dup error in"=w117:errorcluster)  [unwired: 8 in, 1 out]
      }
    }
    frame Error {
      # "Synchronize Caller Events.vi will inform Start Module.vi that the module has launched and will let the code calling Start Module.vi register for broadcasts and would permit the caller receive the broadcast that an error occurred at launch time."
      n149 = call-dynamic "Delacor_lib_QMH_Release Message Queue.vi"("error in (no error)"=w329, "Message Queue"=w327) -> ("error out"=w328:errorcluster)  [unwired: 9 in]
      n150 = call "Synchronize Caller Events.vi"("Singleton Module Admin in"=w330) -> ("error out"=w335:errorcluster)  [unwired: 9 in, 1 out]
      n151 = call "Module Name--constant.vi"() -> ("Module Name"=w333:string)  [unwired: 11 in]
      n152 = Format Into String(format string="An error occurred during initialization. %s is no longer running.", w333) -> (resulting string=w331:string)  [unwired: 2 in, 1 out]
      n153 = Merge Errors(w328, w335) -> (w336:errorcluster)
      n154 = call "Error Reported.vi"("Additional Information"=w331, "Error"=w336) -> ()  [unwired: 9 in, 1 out]
    }
  }
  n155 = Merge Errors(w14, w17) -> (w13:errorcluster)
  n156 = call "Close Module.vi"("error in (no error)"=w13, "Module Admin in"=w8) -> ("error out"=w15:errorcluster, "External Launch"=w1:bool, "Module Admin out"=w2:refnum<class "Delacor_lib_QMH_Module Admin.lvclass">)  [unwired: 7 in]
  n157 = Unregister For Events(event registration refnum=w7, error in=w15) -> (error out=w12:errorcluster)
  "error out" <- w12
  n158 = case "External Launch?" shown="True" w1 {
    tunnel: w12 -> [_ w337]
    frame False {
    }
    frame True {
      n159 = case shown="No Error" w337 {
        frame No Error {
          n160 = invoke class="VI" method="FP.Close"() -> ()  [unwired: 3 in, 3 out]
        }
        frame Error {
          n161 = invoke class="VI" method="FP.Open"("Activate"=TRUE ("Activate?")) -> ()  [unwired: 4 in, 5 out]
        }
      }
    }
  }
  n162 = local write "Module Admin"(w2) -> ()
